vi "Commit Build Settings.vi"(8 "error in (no error)":errorcluster, 11 "DSDIST in":refnum<class "NI_AB_API_DSDIST.lvclass">) -> (0 "error out":errorcluster, 3 "DSDIST out":refnum<class "NI_AB_API_DSDIST.lvclass">)   [LabVIEW 2020, in "NI_AB_API_DSDIST.lvclass"]
uses:
  <vilib>/AppBuilder/AB_API/DSDIST/NI_AB_API_DSDIST.lvclass
  <vilib>/AppBuilder/AB_API/DSDIST/NI_AB_API_DSDIST.lvclass/NI_AB_API_DSDIST.ctl
  <vilib>/AppBuilder/AB_API/SDIST/NI_AB_API_SDIST.lvclass
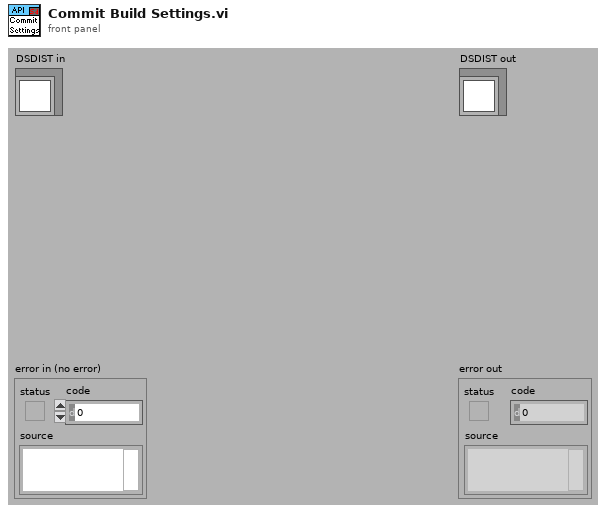
[diagram p1: front panel]
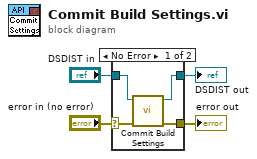
[diagram p0: block diagram]
diagram:
  n1 = case shown="No Error" "error in (no error)" {
    selector: "error in (no error)" -> [w5 w10]
    tunnel: [w6 w10] -> w3
    tunnel: [w7 w9] -> w1
    tunnel: "DSDIST in" -> [w8 w9]
    frame No Error {
      n2 = call-parent "Commit Build Settings.vi"("error in (no error)"=w5, "SDIST in"=w8) -> ("error out"=w6:errorcluster, "SDIST out"=w7:refnum<class "NI_AB_API_DSDIST.lvclass">)  [unwired: 8 in]
    }
    frame Error {
    }
  }
  "error out" <- w3
  "DSDIST out" <- w1
